vi "Button Pressed.vi"(8 "error in (no error)":errorcluster, 10 "selected Option":string, 11 "Module ID":i32=-1) -> (0 "error out":errorcluster)   [LabVIEW 2019, in "Menu Module.lvlib"]
doc: "This will give the Selected Option\n_____\nCreated using Delacor QMH Event Scripter 5.0.0.112."
uses:
  Menu Module.lvlib
  Button Pressed Argument--cluster.ctl
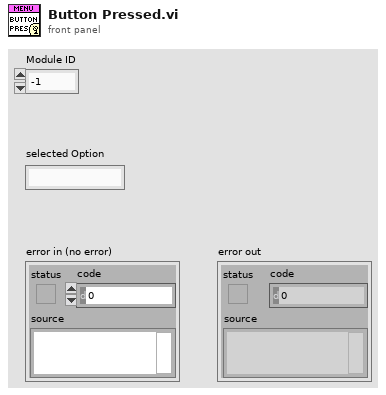
[diagram p1: front panel]
types:
  T1 = typedef "Menu Module.lvlib/Button Pressed Argument--cluster.ctl" = cluster{"Module ID":i32, "selected Option":string}
  T2 = typedef "Menu Module.lvlib/Broadcast Events--cluster.ctl" = cluster{"Module Did Init":refnum<user-event>, "Status Updated":refnum<user-event>, "Error Reported":refnum<user-event>, "Module Did Stop":refnum<user-event>, "Update Module Execution Status":refnum<user-event>, "Button Pressed":refnum<user-event>}
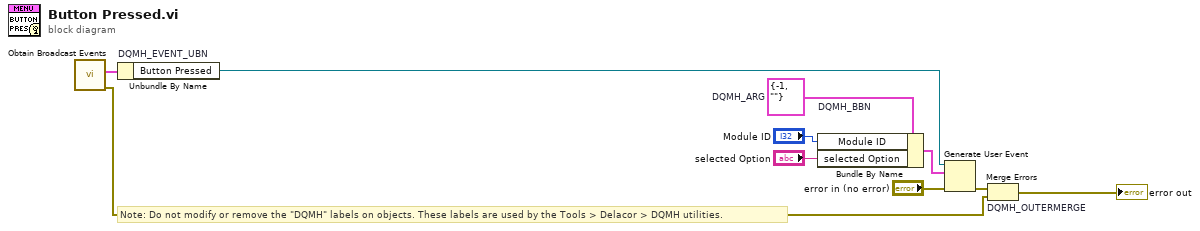
[diagram p0: block diagram]
diagram:
  w5 = T1 {"Module ID"=-1, "selected Option"=""}  # DQMH_ARG
  # "Note: Do not modify or remove the \"DQMH\" labels on objects. These labels are used by the Tools > Delacor > DQMH utilities."
  n1 = call "Obtain Broadcast Events.vi"() -> ("error out"=w2:errorcluster, "Menu Module Broadcast Events"=w1:T2)  [unwired: 10 in]
  n2 = Unbundle By Name "DQMH_EVENT_UBN"(w1) -> ("Button Pressed"=w7:refnum<user-event>)
  n3 = Bundle By Name "DQMH_BBN"(cluster=w5, "Module ID"="Module ID", "selected Option"="selected Option") -> (w8:T1)
  n4 = Generate User Event(user event=w7, event data cluster=w8, error in="error in (no error)") -> (error out=w6:errorcluster)  [unwired: 1 in, 1 out]
  n5 = Merge Errors "DQMH_OUTERMERGE"(w6, w2) -> (→"error out":errorcluster)
